vi "DisatanceFormulA.vi"(10 "B":dbl[](array[numeric]), 11 "A":dbl[](array[numeric])) -> (3 "Distance":dbl)   [LabVIEW 2014]
doc: "Computes the distance between two points. To calculate the distance between a point and the origin, do not connect input B."
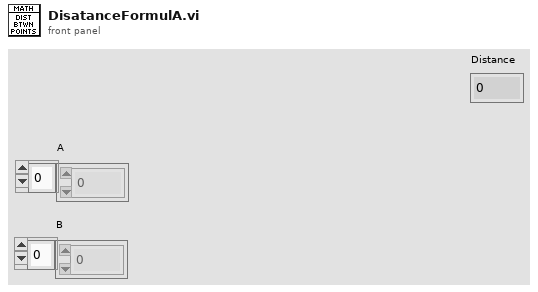
[diagram p1: front panel]
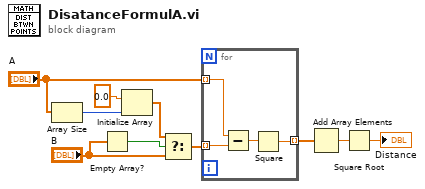
[diagram p0: block diagram]
diagram:
  n1 = Array Size(array="A") -> (size(s)=w7:i32)
  n2 = Empty Array?(array="B") -> (empty?=w4:bool)
  n3 = Initialize Array(0.0 ("element"), w7) -> (w3:dbl[])
  n4 = Select(t=w3, s=w4, f="B") -> (s? t:f=w1:dbl[])
  n5 = for {
    tunnel: "A" -> [w14] mode=indexing
    tunnel: w1 -> [w13] mode=indexing
    tunnel: [w11] -> w10 mode=indexing
    n6 = Subtract(x=w14, y=w13) -> (x-y=w12:dbl)
    n7 = Square(x=w12) -> (x^2=w11:dbl)
  }
  n8 = Add Array Elements(numeric array=w10) -> (sum=w9:dbl)
  n9 = Square Root(x=w9) -> (sqrt(x)=→"Distance":dbl)
